vi "TestSerial.vi"() -> ()   [LabVIEW 2013]
uses:
  <vilib>/Instr/_visa.llb/VISA Configure Serial Port (Instr).vi
panel:
  in  "stop":bool
  out "read buffer":string
  out "Read error":errorcluster
  out "Flush error":errorcluster
  out "Buffer size error":errorcluster
  out "Configure error":errorcluster
  in  "error in (no error)":errorcluster
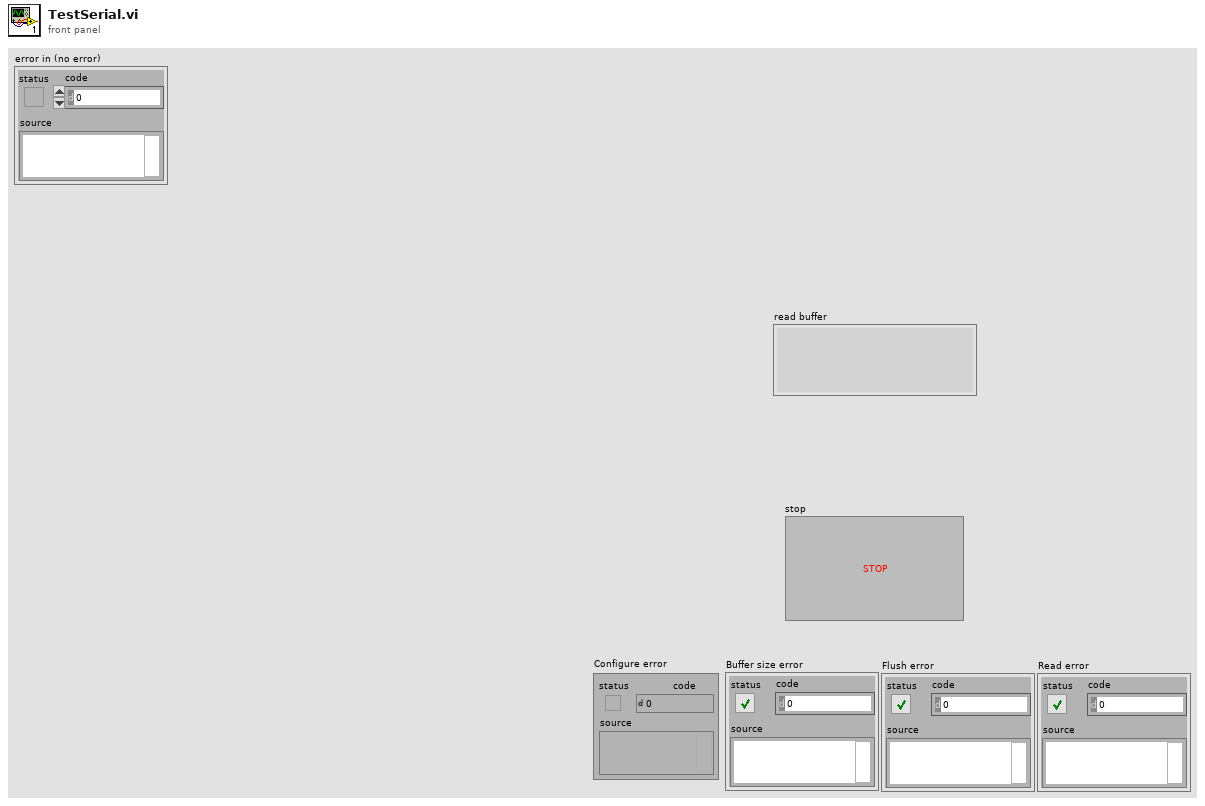
[diagram p1: front panel]
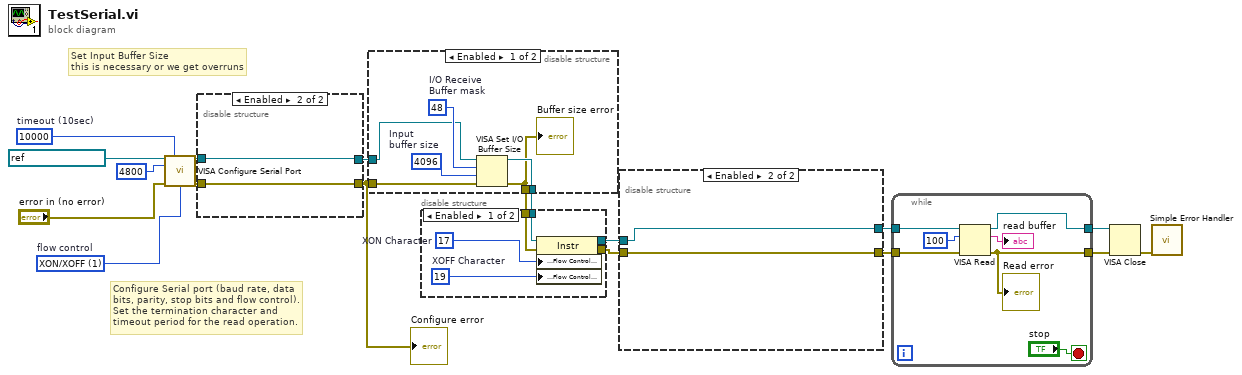
[diagram p0: block diagram]
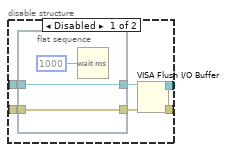
[diagram p2: hidden frame]
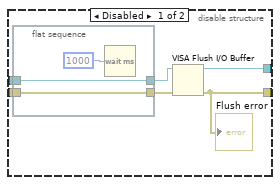
[diagram p5: hidden frame]
diagram:
  w14 = u32 10000  # timeout (10sec)
  w17 = u16 1 items=["None"=0, "XON/XOFF"=1, "RTS/CTS"=2, "DTR/DSR"=4]  # flow control
  # "Set Input Buffer Size\nthis is necessary or we get overruns"
  # "Configure Serial port (baud rate, data\nbits, parity, stop bits and flow control).\nSet the termination character and\ntimeout period for the read operation."
  n1 = call-poly "VISA Configure Serial Port"("VISA resource name"=refnum<visa-resource-name> "ASRL1::INSTR" ("VISA Refnum in"), "timeout (10sec)"=w14, "baud rate (9600)"=u32 4800 ("baud rate"), "error in (no error)"="error in (no error)", "flow control (0:none)"=w17) -> ("VISA resource name out"=w4:refnum<visa-resource-name>, "error out"=w3:errorcluster)  [unwired: 9 in]
  n2 = disable-structure shown="Enabled" {
    disable-tunnel: w4 -> [w24 w29]
    disable-tunnel: w3 -> [w23 w28]
    disable-tunnel: [w20 w29] -> w2
    disable-tunnel: [w19 w28] -> w1
    frame Disabled {
      n3 = flat-sequence {
        tunnel: w24 -> [w26]
        tunnel: [w26] -> w22
        tunnel: w23 -> [w25]
        tunnel: [w25] -> w21
        frame #0 {
          n4 = Wait (ms)(milliseconds to wait=u32 1000) -> ()  [unwired: 1 out]
        }
      }
      n5 = VISA Flush I/O Buffer(VISA resource name=w22, error in (no error)=w21) -> (VISA resource name out=w20:refnum<visa-resource-name>, error out=w19:errorcluster)  [unwired: 1 in]
    }
    frame Enabled {
    }
  }
  "Configure error" <- w1
  n6 = disable-structure shown="Enabled" {
    disable-tunnel: [w34 w37] -> w16
    disable-tunnel: [w33 w36] -> w15
    disable-tunnel: w2 -> [w31 w37]
    disable-tunnel: w1 -> [w30 w36]
    frame Enabled {
      w35 = u32 4096  # Input buffer size
      w32 = u16 48  # I/O Receive Buffer mask
      n7 = VISA Set I/O Buffer Size(VISA resource name=w31, mask (16)=w32, size (4096)=w35, error in (no error)=w30) -> (VISA resource name out=w34:refnum<visa-resource-name>, error out=w33:errorcluster)
      "Buffer size error" <- w33
    }
    frame Disabled {
    }
  }
  n8 = disable-structure shown="Enabled" {
    disable-tunnel: w16 -> [w43 w45]
    disable-tunnel: w15 -> [w42 w44]
    disable-tunnel: [w39 w45] -> w11
    disable-tunnel: [w38 w44] -> w10
    frame Enabled {
      w40 = u8 19  # XOFF Character
      w41 = u8 17  # XON Character
      n9 = property class="Instr"(reference=w43, error in=w42, "Serial Settings:Flow Control XON Character"=w41, "Serial Settings:Flow Control XOFF Character"=w40) -> (reference out=w39:refnum<visa-resource-name>, error out=w38:errorcluster)
    }
    frame Disabled {
    }
  }
  n10 = disable-structure shown="Enabled" {
    disable-tunnel: w11 -> [w51 w56]
    disable-tunnel: w10 -> [w50 w55]
    disable-tunnel: [w47 w56] -> w9
    disable-tunnel: [w46 w55] -> w8
    frame Disabled {
      n11 = flat-sequence {
        tunnel: w51 -> [w53]
        tunnel: [w53] -> w48
        tunnel: w50 -> [w52]
        tunnel: [w52] -> w49
        frame #0 {
          n12 = Wait (ms)(milliseconds to wait=u32 1000) -> ()  [unwired: 1 out]
        }
      }
      n13 = VISA Flush I/O Buffer(VISA resource name=w48, error in (no error)=w49) -> (VISA resource name out=w47:refnum<visa-resource-name>, error out=w46:errorcluster)  [unwired: 1 in]
      "Flush error" <- w46
    }
    frame Enabled {
    }
  }
  n14 = while {
    tunnel: w9 -> [w63]
    tunnel: w8 -> [w62]
    tunnel: [w60] -> w6
    tunnel: [w59] -> w7
    stop <- "stop" stop-if-true
    n15 = VISA Read(VISA resource name=w63, byte count=u32 100, error in (no error)=w62) -> (VISA resource name out=w59:refnum<visa-resource-name>, read buffer=→"read buffer":string, error out=w60:errorcluster)  [unwired: 1 out]
    "Read error" <- w60
  }
  n16 = VISA Close(VISA resource name=w7, error in (no error)=w6) -> (error out=w5:errorcluster)
  n17 = call <vilib>:"Simple Error Handler.vi"("error in (no error)"=w5) -> ()  [unwired: 4 in, 5 out]
